vi "Tosca-Send Error Message.vi"(11 "error in (no error)":errorcluster) -> ()   [LabVIEW 2020]
uses:
  Tosca-Message.ctl
  Tosca-Message Action.ctl
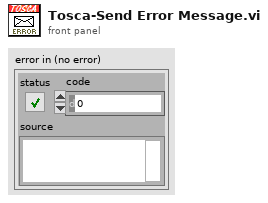
[diagram p1: front panel]
types:
  T1 = typedef "Tosca-Message Action.ctl" = enum16{"None", "Update", "Events", "Timeout", "Error", "Abort"}
  T2 = typedef "Tosca-Message.ctl" = cluster{"Action":T1, "Time":u32, "State":i32, "Events":bool[], "Error":errorcluster}
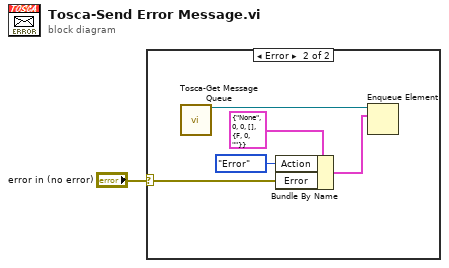
[diagram p0: block diagram]
diagram:
  n1 = case shown="Error" "error in (no error)" {
    selector: "error in (no error)" -> [_ w2]
    frame No Error {
    }
    frame Error {
      n2 = call "Tosca-Get Message Queue.vi"() -> ("Message Queue"=w6:refnum<queue>)  [unwired: 14 in, 1 out]
      n3 = Bundle By Name(cluster=T2 {"Action"=enum."None", "Time"=0, "State"=0, "Events"=[], "Error"={"status"=FALSE, "code"=0, "source"=""}} ("element"), "Action"=Tosca-Message_Action."Error", "Error"=w2) -> (w3:T2)
      n4 = Enqueue Element(queue=w6, element=w3) -> ()  [unwired: 2 in, 3 out]
    }
  }
